vi "DSF.Memory.Cache.Plugin.Get Transfer Cache.vi"(8 "error in (no error)":errorcluster, 10 "Transfer ID":i32, 11 "Plugin Cache in":refnum<class "DSF.Memory.Cache.Plugin.lvclass">) -> (0 "error out":errorcluster, 2 "Transfer Cache":refnum<class "DSF.Memory.Cache.Transfer.lvclass">, 3 "Plugin Cache out":refnum<class "DSF.Memory.Cache.Plugin.lvclass">)   [LabVIEW 2016, in "DSF.Memory.lvlib" / "DSF.Memory.Cache.Plugin.lvclass"]
uses:
  DSF.Memory.Cache.Plugin.lvclass
  DSF.Memory.Cache.Transfer.lvclass
  DSF.Memory.Cache.Plugin.lvclass/DSF.Memory.Cache.Plugin.ctl
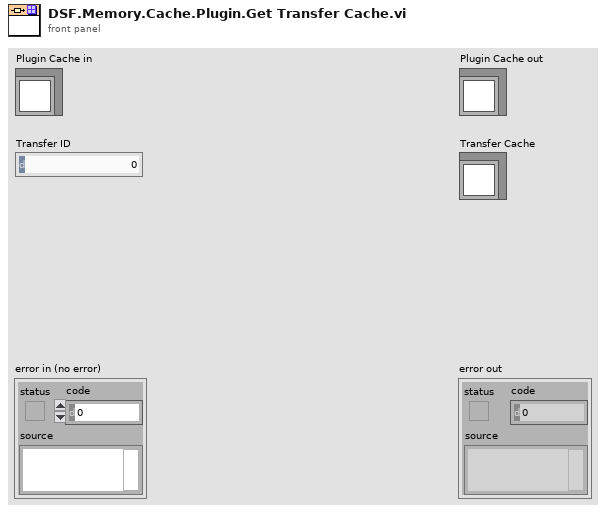
[diagram p1: front panel]
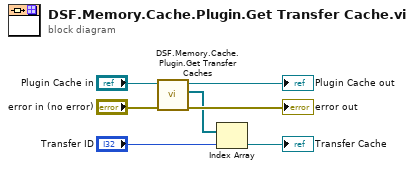
[diagram p0: block diagram]
diagram:
  n1 = call "DSF.Memory.Cache.Plugin.Get Transfer Caches.vi"("error in (no error)"="error in (no error)", "Plugin Cache in"="Plugin Cache in") -> ("error out"=→"error out":errorcluster, "Transfer Caches"=w2:refnum<class "DSF.Memory.Cache.Transfer.lvclass">[], "Plugin Cache out"=→"Plugin Cache out":refnum<class "DSF.Memory.Cache.Plugin.lvclass">)  [unwired: 7 in]
  n2 = Index Array(array=w2, index="Transfer ID") -> (element=→"Transfer Cache":refnum<class "DSF.Memory.Cache.Transfer.lvclass">)
